vi "UpdateClassTemplate.vi"(0 "ClassWriterIn":refnum<class "ClassWriter.lvclass">, 1 "LVClassLibraryRef":refnum<vi>, 2 "ProgressBar":refnum<vi>, 5 "error in (no error)":errorcluster) -> (14 "ClassWriterOut":refnum<class "ClassWriter.lvclass">, 19 "error out":errorcluster)   [LabVIEW 2020, in "ClassWriter.lvclass"]
uses:
  <resource>/Framework/Providers/Open_GDS/ClassProviders/Provider_BaseClassInterface/ClassWriter_class/ClassWriter.lvclass
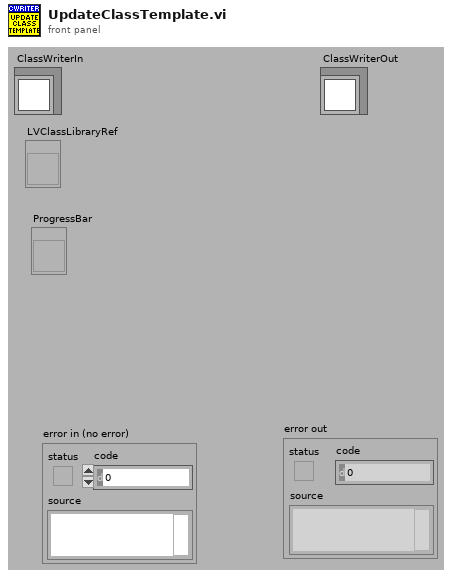
[diagram p1: front panel]
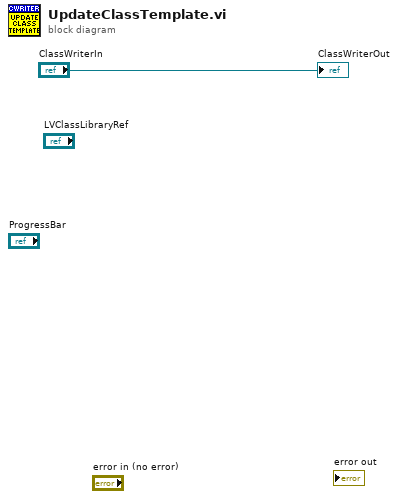
[diagram p0: block diagram]
diagram:
  "ClassWriterOut" <- "ClassWriterIn"
